vi "izmer1.vi"() -> ()   [LabVIEW 2010]
uses:
  70user.lib/TheSigTab.vi
panel:
  in  "filter":bool caption="Фильтр\nперекрёстных помех"
  out "Tper":dbl caption="общая"
  in  "Loop":bool caption="Зациклить данные"
  in  "SaveNow":bool caption="Однократно"
  in  "SaveTime":dbl=1.0 caption="мин" min=1.0 max=120.0
  out "ExtDev":bool caption="Выносной модуль"
  in  "AcqureTime":dbl caption="опроса" format="%#.3g"
  out "Slide":u8(slide) scale=0.0..100.0
  in  "m_s":u16(ring) items=["мин", "сек"]
  in  "Table":string[][](table) caption="Результаты измерений"
  in  "CurvesToo":bool caption="Сохранять графики"
  in  "Continuosly":bool caption="Периодически"
  in  "ScopeToo":bool caption="Сохранять осциллограммы"
  out "Current time":timestamp caption="Время и Дата" format="%<%X\n%x>T"
  in  "Stop":bool
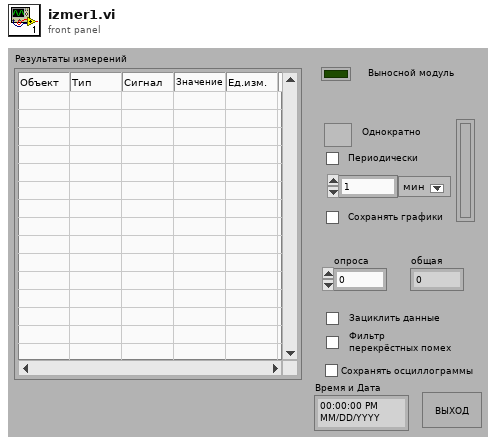
[diagram p1: front panel]
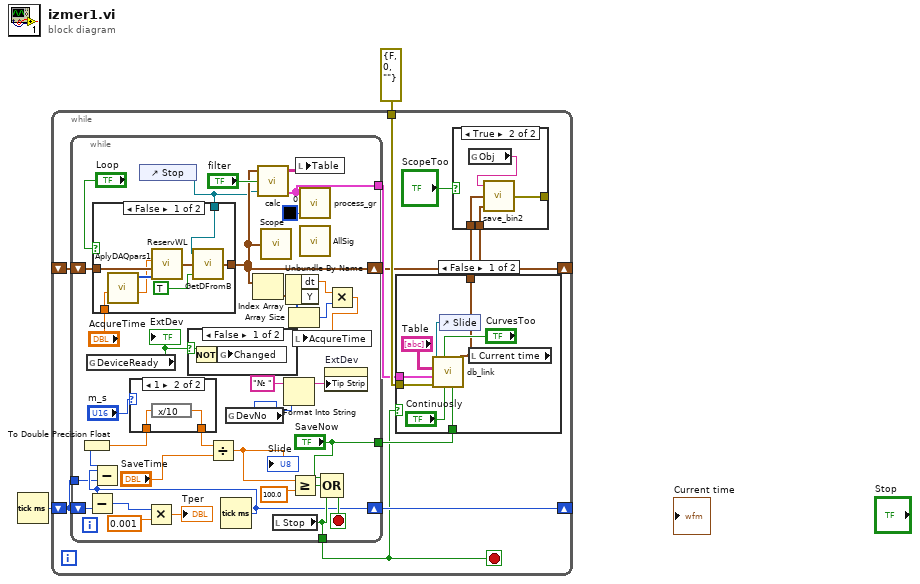
[diagram p0: block diagram]
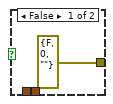
[diagram p2: hidden frame]
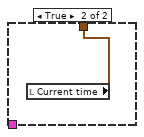
[diagram p3: hidden frame]
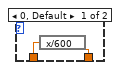
[diagram p4: hidden frame]
diagram:
  n1 = Tick Count (ms)() -> (millisecond timer value=w2:u32)
  n2 = while {
    shift-right: [w12] -> _
    shift-left: w2 -> [w9]
    shift-right: [w5] -> _
    shift-left: _ -> [w11]
    tunnel: errorcluster {"status"=FALSE, "code"=0, "source"=""} ("error out") -> [w10]
    stop <- w6 stop-if-true
    n3 = while {
      shift-right: [w39] -> w5
      shift-left: w11 -> [w58]
      shift-right: [w53] -> w12
      shift-left: w9 -> [w59]
      tunnel: [w55] -> w6
      tunnel: w9 -> [w52]
      tunnel: ["SaveNow"] -> w8
      tunnel: [w45] -> w7
      stop <- w54 stop-if-true
      n4 = global read "TheSigTab.vi" "DeviceReady"() -> (w50:bool)
      "ExtDev" <- w50
      n5 = control-ref of="Stop"() -> (w33:refnum<vi>)
      n6 = case shown="False" "Loop" {
        tunnel: w58 -> [w75 w76]
        tunnel: [w72 w76] -> w39
        tunnel: "AcqureTime" -> [w69 _]
        tunnel: w33 -> [w68 _]
        frame False {
          n7 = call "AplyDAQpars1.vi"("AcqTimeIn"=w69) -> ("t1-t0"=w70:dbl, "Idxs"=w74:i32[])  [unwired: 5 in]
          n8 = call "ReservWL.vi"("Tags"=w74, "ArrayIn"=w75, "t1-t0"=w70) -> ("Array"=w73:waveform(i16)[])  [unwired: 1 in]
          n9 = call "GetDFromB.vi"("Control"=TRUE, "ArrayIn"=w73, "Bool Refnum"=w68) -> ("ArrayOut"=w72:waveform(i16)[])
        }
        frame True {
        }
      }
      n10 = case shown="False" w50 {
        selector: w50 -> [w67 _]
        frame False {
          n11 = Not(x=w67) -> (.not. x?=w66:bool)
          n12 = global write "TheSigTab.vi" "Changed"(w66) -> ()
        }
        frame True {
        }
      }
      n13 = Tick Count (ms)() -> (millisecond timer value=w53:u32)
      n14 = Subtract(x=w53, y=w59) -> (x-y=w49:u32)
      n15 = Subtract(x=w53, y=w52) -> (x-y=w51:u32)
      n16 = To Double Precision Float(number=w51) -> (double precision float=w28:dbl)
      n17 = case shown="1" "m_s" {
        tunnel: w28 -> [w63 w65]
        tunnel: [w62 w64] -> w27
        frame 0, Default {
          n18 = expression code="x/600"(w63) -> (w62:dbl)
        }
        frame 1 {
          n19 = expression code="x/10"(w65) -> (w64:dbl)
        }
      }
      n20 = Multiply(x=w49, y=0.001 ("x")) -> (x*y=→"Tper":dbl)
      n21 = Divide(x=w27, y="SaveTime") -> (x/y=w43:dbl)
      "Slide" <- w43
      n22 = global read "TheSigTab.vi" "DevNo"() -> (w30:u32)
      n23 = Index Array(array=w39) -> (element=w38:waveform(i16))  [unwired: 1 in]
      n24 = call "calc.vi"("Acquire"=w33, "filter"="filter", "ArrayIn"=w39) -> ("AllMeasures"=w45:cluster{"x0":dbl, "dx":dbl, "y":sgl[][]}[], "Values"=w61:string[][])  [unwired: 1 in]
      n25 = call "Scope.vi"("Array"=w39) -> ()
      n26 = local read "Stop"() -> (w55:bool)
      n27 = Format Into String(initial string="№ ", w30) -> (resulting string=w32:string)  [unwired: 2 in, 1 out]
      n28 = Unbundle By Name(w38) -> ("dt"=w36:dbl, "Y"=w37:i16[])
      n29 = Array Size(array=w37) -> (size(s)=w35:i32)
      n30 = Greater Or Equal?(x=w43, y=100.0 ("x")) -> (x >= y?=w40:bool)
      n31 = local write "Table"(w61) -> ()
      n32 = call "process_gr.vi"("Color Box"=u32 0, "AllMeasures"=w45) -> ()  [unwired: 2 in, 2 out]
      n33 = call "AllSig.vi"() -> ()  [unwired: 1 in]
      n34 = Compound Arithmetic op=OR("SaveNow", w40, w55) -> (w54:bool)
      n35 = property on="ExtDev" class="Bool (strict)"("Tip Strip"=w32) -> ()  [unwired: 2 in, 2 out]
      n36 = Multiply(x=w36, y=w35) -> (x*y=w34:dbl)
      n37 = local write "AcqureTime"(w34) -> ()
    }
    n38 = case shown="False" w6 {
      tunnel: w10 -> [w25 _]
      tunnel: w8 -> [w24 _]
      tunnel: w7 -> [w22 _]
      tunnel: [w18 w26] -> w4
      frame False {
        n39 = control-ref of="Slide"() -> (w21:refnum<vi>)
        n40 = local read "Current time"() -> (w18:timestamp)
        n41 = call "db_link.vi"("Current time"=w18, "SaveNow"=w24, "Continuosly"="Continuosly", "SaveCurves?"="CurvesToo", "error in"=w25, "AllMeasures"=w22, "Table"="Table", "reference"=w21) -> ()  [unwired: 3 in, 1 out]
      }
      frame True {
        n42 = local read "Current time"() -> (w26:timestamp)
      }
    }
    n43 = case shown="True" "ScopeToo" {
      tunnel: [errorcluster {"status"=FALSE, "code"=0, "source"=""} ("error out") w17] -> _
      tunnel: w5 -> [_ w16]
      tunnel: w4 -> [_ w15]
      frame False {
      }
      frame True {
        n44 = global read "TheSigTab.vi" "Obj"() -> (w14:string)
        n45 = call "save_bin2.vi"("ArrayOut"=w16, "Current time"=w15, "Object"=w14) -> ("error out"=w17:errorcluster)
      }
    }
  }
